vi "GUI_Bella_Control_Center_iP2.vi"() -> ()   [LabVIEW 2020]
uses:
  Shared/GUI_Template/GUI_master/tcp_new_data_event.ctl
  Shared/GUI_Template/GUI_master/tcp new data cluster.ctl
  GUI_TestStand/Fire button.ctl
  Device Drivers/DG645/subVIs/TriggerSource_TypDef.ctl
  <vilib>/Utility/config.llb/Write Key (I32).vi
  <vilib>/Platform/browser.llb/Open URL in Default Browser (string).vi
  <vilib>/Utility/config.llb/NI_LVConfig.lvlib
panel:
  out "got manpar ofi bool data":bool
  out "got manpar ofi data":bool
  out "set expt editor":bool
  in  "Delay.Ch D::10":dbl=-1.631e-06 caption="Delay D" min=-0.1 max=20.0 format="%.4f"
  in  "value6::42":dbl=0.006 caption="PostScanRate" min=0.1 max=1.0 format="%#_3f"
  in  "value5::42":dbl=0.006 caption="1BL-2BL-\nSplitter-Rpcnt" min=-9999999.0 max=9999999.0 format="%#_6p"
  in  "value6::43":bool=TRUE caption="GhostFoil-In"
  in  "value5::43":bool=TRUE caption="1BL-Energy\nMeter-In"
  in  "value4::43":bool=TRUE caption="2BLFoil-In"
  in  "value3::43":bool=TRUE caption="1BLFoil-In"
  in  "value2::43":bool=TRUE caption="ClunkerIn"
  out "CurrentStatus":string
  in  "MoveStage":bool
  in  "Position.Ch1::44":dbl caption="Current Position" min=0.0 max=150.0
  in  "GUIdevice 44":string="STAGE-LT-Megattenuator"
  in  "GUIdevice 43":string="MANPAR-BELLA-OFI-Boolean"
  in  "GUIdevice 42":string="MANPAR-BELLA-OFI"
  out "HPD2 to match HPD":dbl
  in  "Save \ncreenshots":bool
  out "error out":errorcluster
  out "HPD - focus":dbl
  in  "value1::42":dbl=230.0 caption="focus on HPD" min=-9999999.0 max=9999999.0
  in  "value0::43":bool=TRUE caption="SCS"
  in  "Thales.DIAG_CU_Output_Percent_1::37":dbl caption="Amp2 att (%)" min=1.0 max=100.0 step=500.0 format="%.2f"
  in  "GUIdevice 37":string="SVE-LT-Thales"
  in  "Scan":T1(ring)
  in  "LogTable":bool
  in  "New Google\nExpLog for new day?":bool=TRUE
  out "standard output":string
  in  "Create Log":bool caption="LogTable"
  in  "Position.Channel 5::31":T2(ring) caption="FROG foil"
  in  "Position.Channel 2::31":T2(ring) caption="Little Rick"
  in  "Step size 2":dbl=20.0 caption="Step size" min=-22.0 max=22.0
  in  "Position.Axis 4::33":dbl caption="Holy M V F4" min=-100000.0 max=100000.0 step=500.0
  in  "Position.Axis 3::33":dbl caption="Holy M H F3" min=-1000000.0 max=1000000.0 step=500.0
  in  "Position.Axis 2::33":dbl caption="Bessel M3 V F2" min=-100000.0 max=100000.0 step=500.0
  in  "Position.Axis 1::33":dbl caption="Bessel M3 H F1" min=-100000.0 max=100000.0 step=500.0
  in  "GUIdevice 33":string="MCD-PL1-picosOFI1"
  in  "GUIdevice 4":string="STAGE-PL1-Capstage1"
  in  "GUIdevice 31":string="1WIRE-BELLA-Flipper"
  in  "Amplitude.Ch GH::10":dbl=-1.631e-06 caption="Shot Shutter V" min=0.5 max=5.0 format="%.1f"
  in  "Rate (Hz)":dbl=0.3
  in  "Heater Alignment Directions":bool
  in  "Position.Axis 3::15":dbl caption="XY" min=-3.0 max=16.0 format="%.4f"
  in  "Position.Axis 2::15":dbl caption="Y" min=-3.0 max=17.0 format="%.4f"
  in  "Position.Axis 1::15":dbl caption="X" min=-3.0 max=13.0 format="%.4f"
  in  "GUIdevice 24":string="STAGE-HEAT-TL1"
  in  "Encoder position::23":dbl caption="position HPD2" min=0.0 max=600.0 format="%.1f"
  in  "position::3":dbl caption="position HPD" min=0.0 max=600.0 format="%.1f"
  in  "GUIdevice 23":string="STAGE-HPD-Far"
  in  "GUIdevice 22":string="MANPAR-BELLA-FireCont"
  in  "Allow Fire Continues":bool
  out "Fire continues Indicator":bool caption="firing"
  in  "Fire Button":T3=TRUE
  in  "Trigger.Source::10":T4 caption="SRS Trigger Mode"
  out "Absolute discharge timing":dbl caption="delay from pk" format="%#.3p"
  in  "Delay.Ch E::17":dbl caption="Timing box" min=-0.1 max=0.1 format="%.3p"
  in  "value0::22":bool caption="Fire continuosly"
  in  "GUIdevice 15":string="MCD-HEAT-ESP1"
  in  "GUIdevice 17":string="DDG-AA-SRS0"
  out "error IO 2":errorcluster
  out "fire::10":string
  out "tcp data event":T5
  in  "UDP error message":string
  in  "GUIdevice 13":string="DDG-AA-SRS2"
  in  "GUIdevice 2":string="MANPAR-BELLA-General"
  in  "GUIdevice 10":string="DDG-AA-ShotCntrl"
  in  "GUIdevice 1":string="HEX-PL1-1"
  in  "GUIdevice 3":string="STAGE-HPD-Tel"
  in  "Position.Axis 1::9":dbl caption="Comp1 Translation" min=-50.0 max=50.0 format="%.3f"
  in  "GUIdevice 9":string="STAGE-1BL-Compression"
  in  "stop":bool
  # "BELLA ip2 CONTROL CENTER"
  # "Scan"
  # "Safety"
  # "needs manpar-bella-ofi on\nMANPAR-BELLA-OFI-Boolean"
  # "Discharge timing (s)"
  # "1wire"
  # "DG"
  # "PICOS"
  # "Heater timing (s)"
  # "HPD Stage"
  # "Megattenuator Stage"
  # "Attenuate"
  # "OUT"
  # "IN"
  # "Compressor"
  # "Heater Alignment"
  # "Heat ESP0"
  # "Heat ESP1"
  # "Heat Pico"
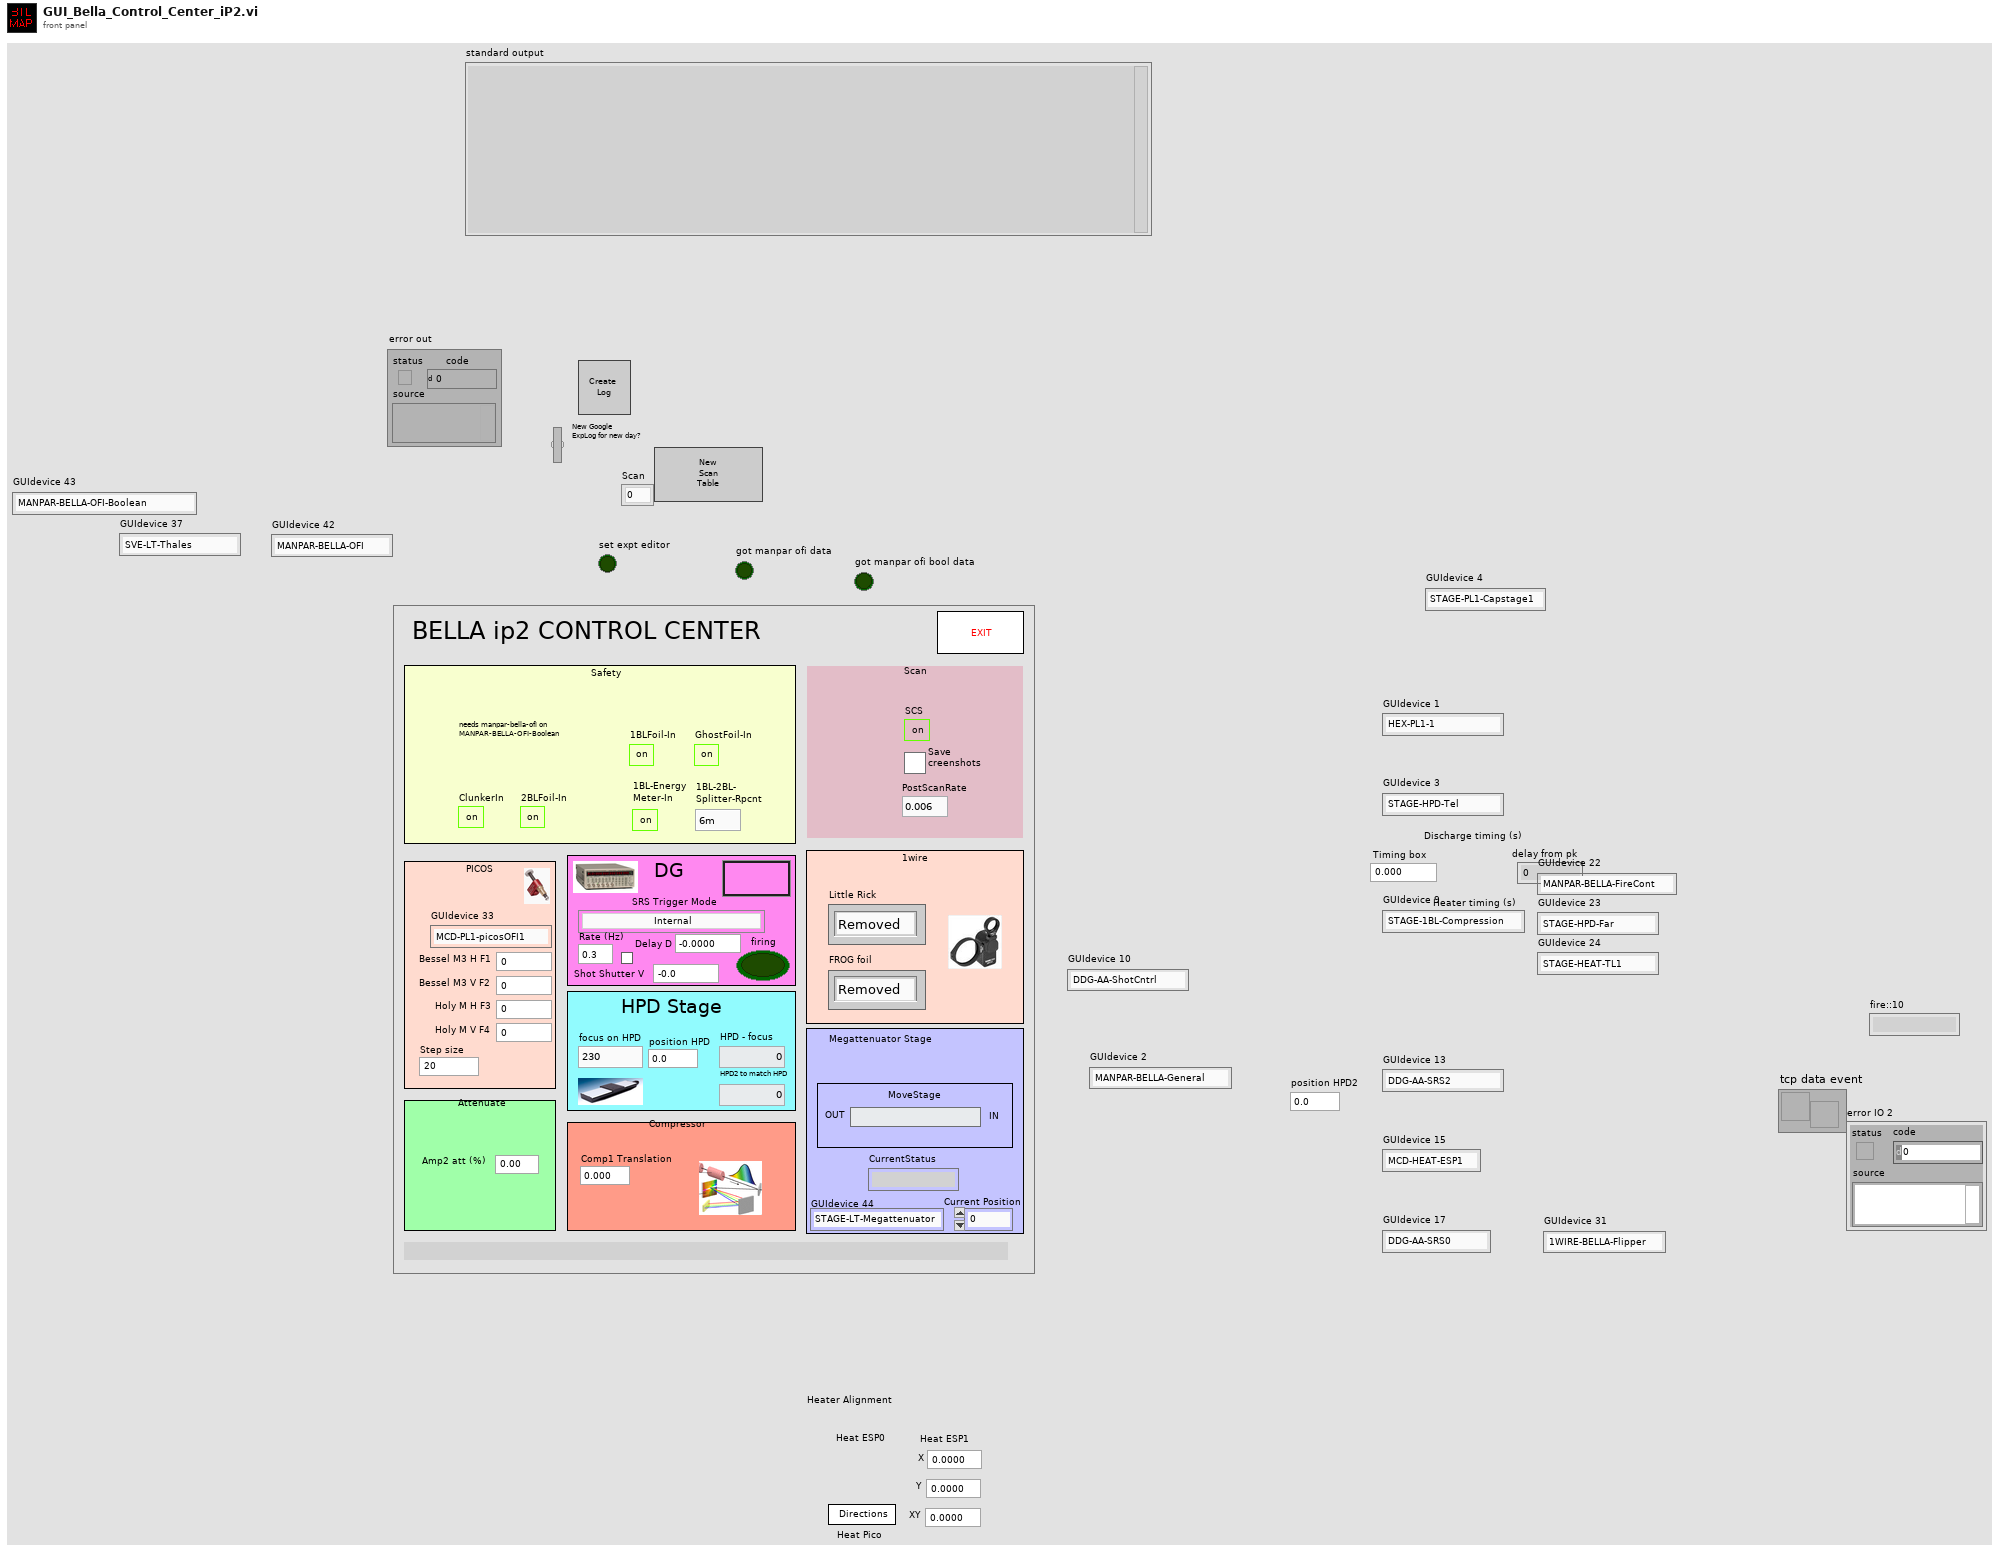
[diagram p1: front panel]
types:
  T1 = enum16{"0", "1", "2", "3", "4", "5", "6", "7", "8", "9", "10", "11", "12", "13", "14", "15", "16", "17", "18", "19", "20", "21", "22", "23", "24", "25", "26", "27", "28", "29", "30", "31", "32", "33", "34", "35", "36", "37", "38", "39", "40", "41", "42", "43", "44", "45", "46", "47", "48", "49", "50", "51", "52", "53", "54", "55", "56", "57", "58", "59", "60", "61", "62", "63", "64", "65", "66", "67", "68", "69", "70", "71", "72", "73", "74", "75", "76", "77", "78", "79", "81", "82", "83", "84", "85", "86", "87", "88", "89", "90", "91", "92", "93", "94", "95", "96", "97", "98", "99", ""}
  T2 = enum16{"Removed", "Inserted", "Unknown", "Moving"}
  T3 = typedef "Fire button.ctl" = bool
  T4 = typedef "TriggerSource_TypDef.ctl" = enum16{"Internal", "External rising edges", "External falling edges", "Single shot external rising edges", "Single shot external falling edges", "Single shot", "Line"}
  T5 = typedef "tcp_new_data_event.ctl" = refnum<user-event>
  T6 = typedef "tcp new data cluster.ctl" = cluster{"EventEnum":enum16{"new data", "connection status update"}, "Device name":string}
  T7 = enum32{"invalid app kind", "Development System", "Run Time System", "Student Edition", "Embedded LabVIEW", "Evaluation", "Custom"}
  T8 = enum32{"Invalid", "Standard", "Closed", "Hidden", "Minimized", "Maximized"}
  T9 = enum8{"Enabled", "Disabled", "Disabled and Grayed Out"}
  T10 = typedef "imagedata.ctl" = cluster{"image type":i32, "image depth":i32, "image":u8[], "mask":u8[], "colors":u32[], "Rectangle":cluster{"left":i16, "top":i16, "right":i16, "bottom":i16}}
  T11 = typedef "NI_LVConfig.lvlib/Config Data RefNum.ctl" = refnum<k1>
  T12 = cluster{"Core":cluster{"Current VI Reference":refnum<vi>, "Close Panel on Exit?":bool}, "Heater timing offset":dbl, "Discharge timing offset":dbl, "Jet trigger":bool, "Tik1":u32, "Tik2":u32, "Fire Continues Allowed":bool}
  T13 = cluster{"Current VI Reference":refnum<vi>, "Close Panel on Exit?":bool}
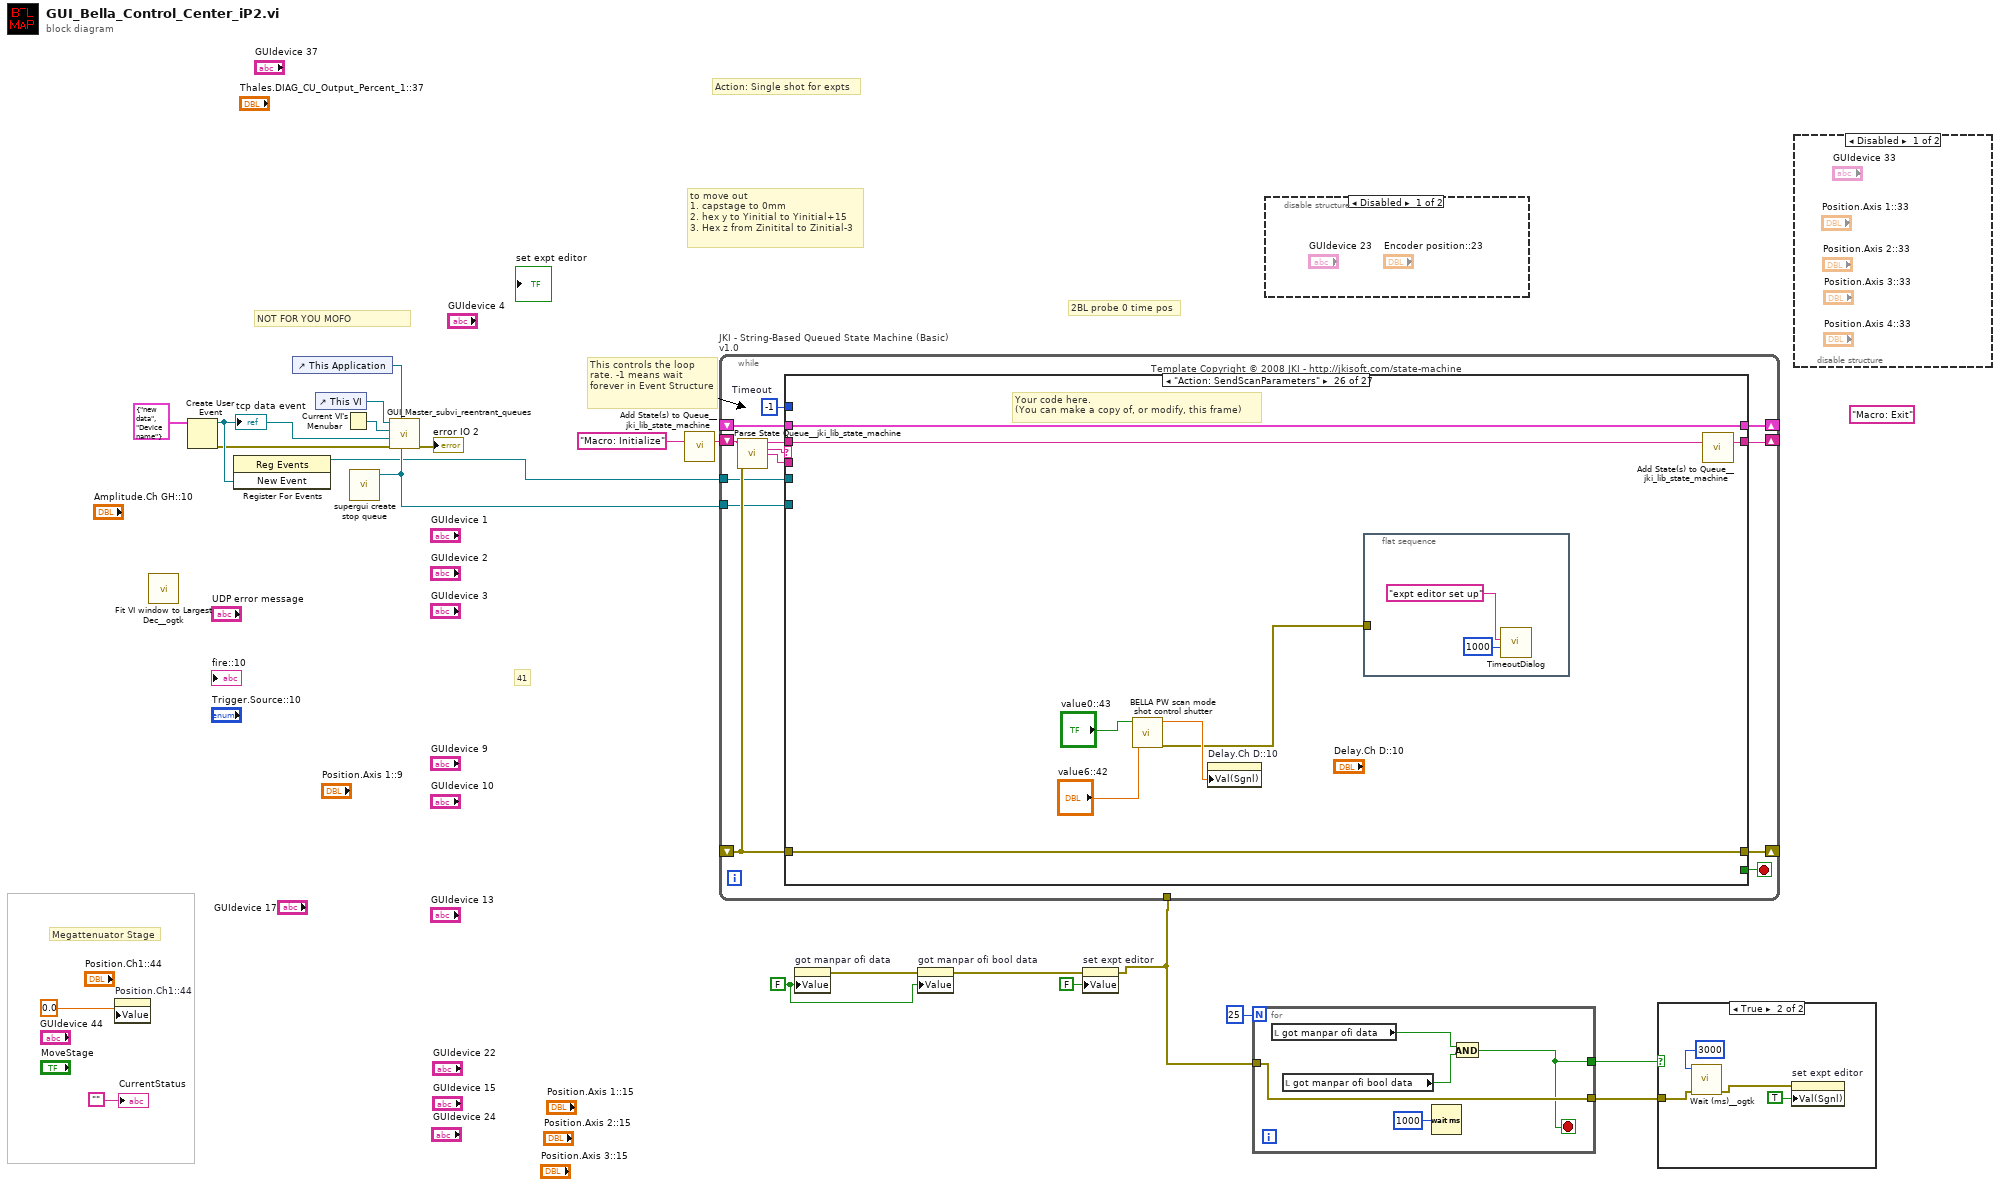
[diagram p0: block diagram]
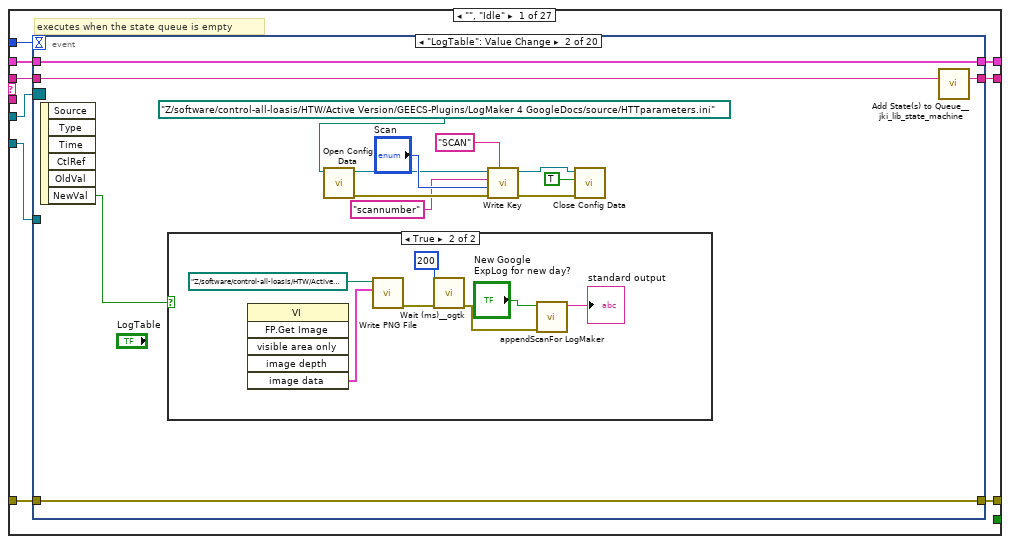
[diagram p5: hidden frame]
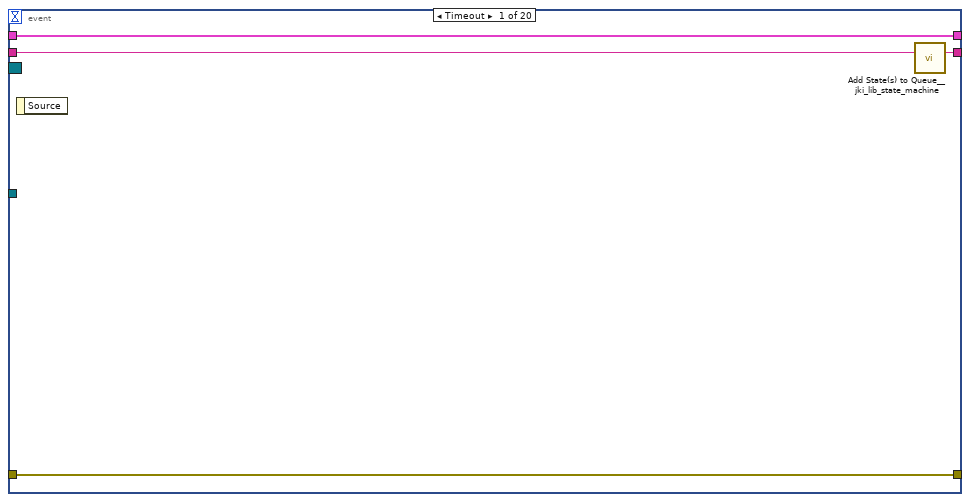
[diagram p6: hidden frame]
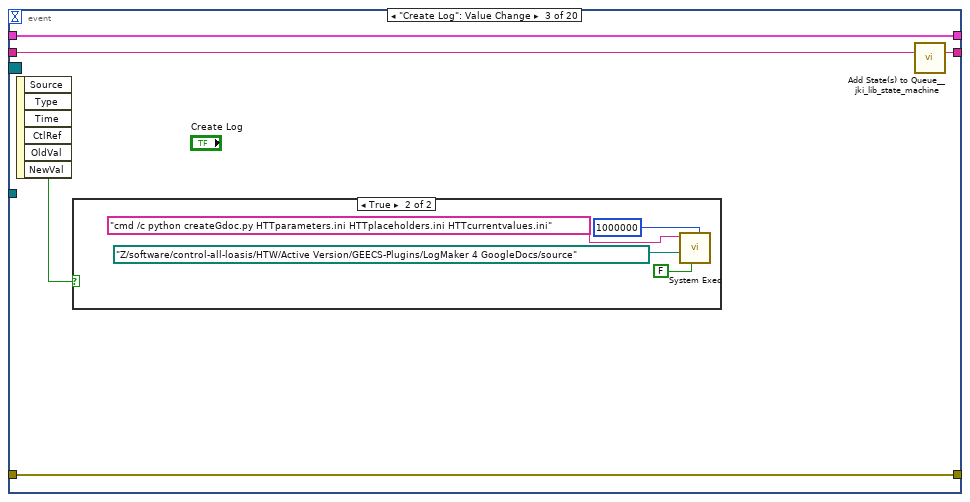
[diagram p8: hidden frame]
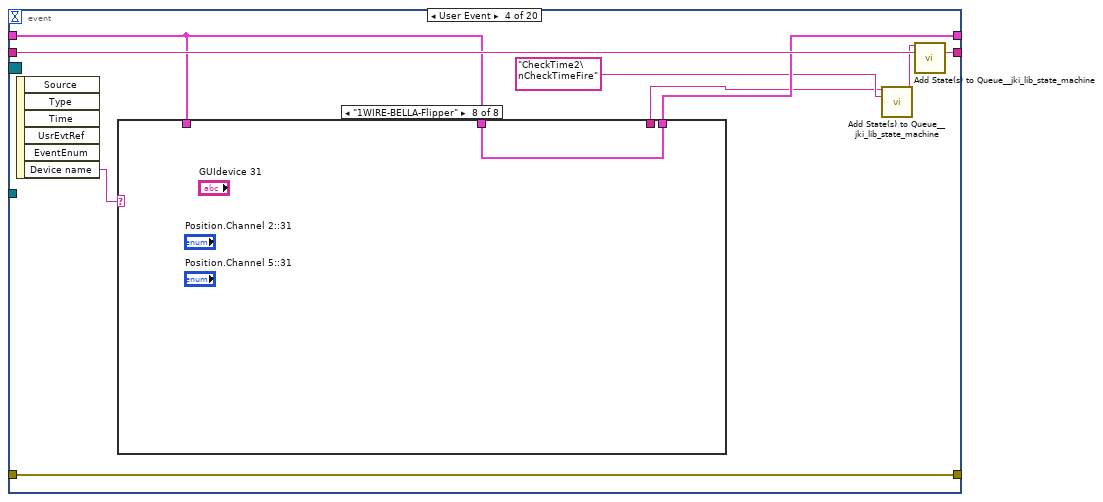
[diagram p10: hidden frame]
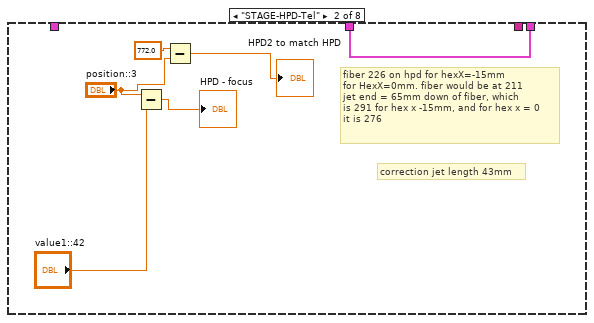
[diagram p12: hidden frame]
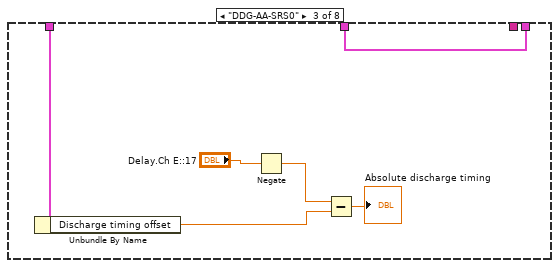
[diagram p13: hidden frame]
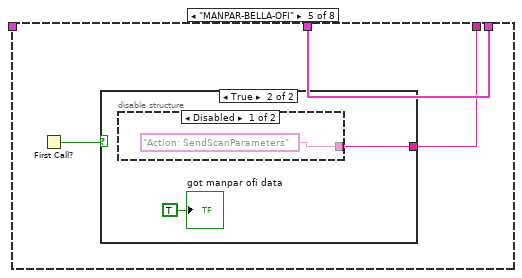
[diagram p15: hidden frame]
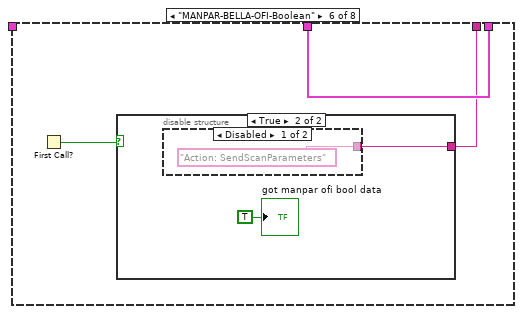
[diagram p18: hidden frame]
diagram:
  w5 = FALSE ("got manpar ofi data")
  (unwired) "Macro: Exit"
  # "41"
  # "Megattenuator Stage"
  # "2BL probe 0 time pos"
  # "Action: Single shot for expts"
  # "to move out\n1. capstage to 0mm\n2. hex y to Yinitial to Yinitial+15\n3. Hex z from Zinitital to Zinitial-3"
  # "This controls the loop rate. -1 means wait forever in Event Structure"
  # "NOT FOR YOU MOFO"
  n1 = property on="Position.Ch1::44" class="DigNum (strict)"("Value"=0.0 ("Position.Ch1::44")) -> ()  [unwired: 2 in, 2 out]
  n2 = call <userlib>:"Fit VI window to Largest Dec__ogtk.vi"() -> ()  [unwired: 6 in, 2 out]
  n3 = Create User Event(user event datatype=T6 {"EventEnum"=enum."new data", "Device name"="Device name"} ("New Event")) -> (user event=w20:refnum<user-event>, error out=w19:errorcluster)  [unwired: 1 in]
  "tcp data event" <- w20
  n4 = register-events(w20) -> (reference out=w11:refnum<event-registration>)  [unwired: 2 in, 1 out]
  n5 = control-ref of="This Application"() -> (w21:refnum<vi>)
  n6 = control-ref of="This VI"() -> (w15:refnum<vi>)
  n7 = Current VI's Menubar() -> (w17:refnum<k9>)
  n8 = call "supergui create stop queue.vi"() -> ("STOP Queue out"=w12:refnum<queue>)  [unwired: 11 in]
  n9 = call "GUI_Master_subvi_reentrant_queues.vi"("STOP Queue in"=w12, "This Application"=w21, "error in (no error)"=w19, "tcp data event"=w20, "Caller menu reference"=w17, "Caller VI ref"=w15) -> ("error out"=→"error IO 2":errorcluster)  [unwired: 5 in]
  n10 = call <vilib>:"Add State(s) to Queue__jki_lib_state_machine.vi"("State(s) in (\"\")"="Macro: Initialize") -> ("States Out"=w13:string)  [unwired: 14 in]
  n11 = property on="got manpar ofi data" class="Bool (strict)"("Value"=w5) -> (error out=w6:errorcluster)  [unwired: 2 in, 1 out]
  n12 = property on="got manpar ofi bool data" class="Bool (strict)"(error in=w6, "Value"=w5) -> (error out=w7:errorcluster)  [unwired: 1 in, 1 out]
  n13 = property on="set expt editor" class="Bool (strict)"(error in=w7, "Value"=FALSE ("set expt editor")) -> (error out=w4:errorcluster)  [unwired: 1 in, 1 out]
  n14 = while "JKI - String-Based Queued State Machine (Basic) v1.0" {
    shift-right: [w27] -> _
    shift-left: _ -> [w26]
    shift-right: [w30] -> _
    shift-left: _ -> [w24]
    shift-right: [w29] -> _
    shift-left: w13 -> [w31]
    tunnel: w11 -> [w23]
    tunnel: w12 -> [w22]
    tunnel: w4 -> [_]
    stop <- w28 stop-if-true
    w25 = -1  # Timeout
    # "Template Copyright © 2008 JKI - http://jkisoft.com/state-machine"
    n15 = call <vilib>:"Parse State Queue__jki_lib_state_machine.vi"("State Queue"=w31, "Error In (no error)"=w24) -> ("Remaining States"=w33:string, "Current State"=w34:string, "Arguments"=w32:string)  [unwired: 11 in]
    n16 = case shown="\"Action: SendScanParameters\"" w34 {
      selector: w34 -> [_ _ w279 _ _ _ _ _ _ _ _ _ _ _ _ _ _ _ _ _ _ _ _ _ _ _ _]
      tunnel: w33 -> [w43 w278 w283 w301 w307 w312 w316 w327 w333 w337 w341 w347 w358 w384 w389 w402 w406 w412 w421 w458 w469 w481 w493 w502 w506 w514 w521]
      tunnel: w32 -> [_ _ _ _ _ _ _ _ _ _ _ w342 w352 _ _ _ _ _ _ _ _ _ _ _ _ _ _]
      tunnel: w26 -> [w41 w275 w281 w292 w304 w310 w313 _ w328 w334 w339 w345 w354 w381 w386 w399 w403 w409 w418 w446 w465 w475 w490 w500 w503 w511 w518]
      tunnel: [w40 w276 w285 w298 errorcluster {"status"=FALSE, "code"=0, "source"=""} ("error out") w309 w314 w324 w329 w335 w338 w343 w355 w382 w387 w400 w404 w410 w419 w456 w463 w470 w491 w497 w504 w512 w519] -> w30
      tunnel: w24 -> [w39 w276 w284 w298 w303 w309 w314 w324 w330 w335 w338 w344 w356 w382 w387 w400 w404 w410 w419 w456 w467 w471 w491 w498 w504 w512 w519]
      tunnel: [w42 w277 w282 w300 w306 w311 w315 w326 w332 w336 w340 w346 w357 w383 w388 w401 w405 w411 w420 w457 w468 w480 w492 w501 w505 w513 w520] -> w29
      tunnel: [_ _ _ _ _ TRUE _ _ _ _ _ _ _ _ _ _ _ _ _ _ _ _ _ _ _ _ _] -> w28
      tunnel: [w35 w275 w281 w299 w304 w310 w313 w325 w328 w334 w339 w345 w354 w381 w386 w399 w403 w409 w418 w455 w465 w474 w489 w500 w503 w511 w518] -> w27
      tunnel: w25 -> [w38 _ _ _ _ _ _ _ _ _ _ _ _ _ _ _ _ _ _ _ _ _ _ _ _ _ _]
      tunnel: w23 -> [w37 _ _ _ _ _ _ _ _ _ _ _ _ _ _ _ _ _ _ _ _ _ _ _ _ _ _]
      tunnel: w22 -> [w36 _ _ _ _ _ _ _ _ _ _ _ _ _ _ w391 _ _ _ _ _ _ _ _ _ _ _]
      frame "", "Idle" {
        # "executes when the state queue is empty"
        n17 = event shown="[1] \"LogTable\": Value Change" {
          selector: w37 -> [_ _ _ _ _ _ _ _ _ _ _ _ _ _ _ _ _ _ _ _]
          dyn-events: _ -> [_ _ _ _ _ _ _ _ _ _ _ _ _ _ _ _ _ _ _ _]
          timeout: w38 -> [_ _ _ _ _ _ _ _ _ _ _ _ _ _ _ _ _ _ _ _]
          tunnel: w43 -> [w47 w61 w73 w86 w122 w124 w129 w139 w149 w159 w169 w179 w188 w196 w205 w229 w239 w246 w248 w274]
          tunnel: [w46 w60 w72 w85 w121 w125 w130 w140 w150 w160 w170 w180 w189 w196 w204 w227 w239 w246 w247 w273] -> w42
          tunnel: w41 -> [w44 w58 w70 w82 w119 w127 w132 w142 w152 w162 w172 w182 w191 w195 w207 w231 w240 w245 w255 w271]
          tunnel: [w45 w59 w71 w84 w120 w126 w131 w141 w151 w161 w171 w181 w190 w193 w210 w230 w238 w244 w254 w272] -> w40
          tunnel: w39 -> [w45 w59 w71 w84 w120 w126 w131 w141 w151 w161 w171 w181 w190 w194 w209 w230 w238 w244 w254 w272]
          tunnel: [w44 w58 w70 w81 w119 w127 w132 w142 w152 w162 w172 w182 w191 w195 w208 w231 w240 w245 w255 w271] -> w35
          tunnel: w36 -> [_ _ _ _ _ _ _ _ _ _ _ _ _ _ _ _ _ _ _ _]
          event Timeout {
            n18 = event-data() -> ()  [unwired: 1 in, 1 out]
            n19 = call <vilib>:"Add State(s) to Queue__jki_lib_state_machine.vi"("State(s) in (\"\")"=w47) -> ("States Out"=w46:string)  [unwired: 14 in]
          }
          event "LogTable": Value Change {
            n20 = event-data() -> ("NewVal"=w48:bool)  [unwired: 1 in, 5 out]
            n21 = case shown="True" w48 {
              frame False {
              }
              frame True {
                n22 = invoke class="VI" method="FP.Get Image"() -> ("image data"=w68:T10)  [unwired: 6 in, 5 out]
                n23 = call <vilib>:"Write PNG File.vi"("image data"=w68, "path to PNG file"=path "Z:/software/control-all-loasis/HTW/Active Version/GEECS-Plugins/LogMaker 4 GoogleDocs/source/frontpanel.png" ("report file path")) -> ("error out"=w63:errorcluster)  [unwired: 8 in, 1 out]
                n24 = call <userlib>:"Wait (ms)__ogtk.vi"("error in (no error)"=w63, "milliseconds to wait"=u32 200 ("millisecond timer value")) -> ("error out"=w62:errorcluster)  [unwired: 8 in, 1 out]
                n25 = call "appendScanFor LogMaker.vi"("error in (no error)"=w62, "New Google\nExpLog for new day?"="New Google\nExpLog for new day?") -> ("standard output"=→"standard output":string)  [unwired: 9 in]
              }
            }
            n26 = call <vilib>:"Open Config Data.vi"("configuration file path"=path "Z:/software/control-all-loasis/HTW/Active Version/GEECS-Plugins/LogMaker 4 GoogleDocs/source/HTTparameters.ini") -> ("error out"=w55:errorcluster, "refnum"=w53:T11)  [unwired: 8 in, 1 out]
            n27 = call-poly <vilib>:"Write Key.vi"("section"="SCAN", "error in (no error)"=w55, "value"="Scan", "key"="scannumber", "refnum"=w53) -> ("error out"=w56:errorcluster, "refnum out"=w54:T11)  [unwired: 4 in, 1 out]
            n28 = call <vilib>:"Close Config Data.vi"("error in (no error)"=w56, "write file if changed (T)"=TRUE, "refnum"=w54) -> ()  [unwired: 7 in, 2 out]
            n29 = call <vilib>:"Add State(s) to Queue__jki_lib_state_machine.vi"("State(s) in (\"\")"=w61) -> ("States Out"=w60:string)  [unwired: 14 in]
          }
          event "Create Log": Value Change {
            n30 = event-data() -> ("NewVal"=w69:bool)  [unwired: 1 in, 5 out]
            n31 = case shown="True" w69 {
              frame False {
              }
              frame True {
                n32 = call <vilib>:"System Exec.vi"("expected output size  (4096)"=u32 1000000, "run minimized? (F)"=FALSE, "working directory"=path "Z:/software/control-all-loasis/HTW/Active Version/GEECS-Plugins/LogMaker 4 GoogleDocs/source", "command line"="cmd /c python createGdoc.py HTTparameters.ini HTTplaceholders.ini HTTcurrentvalues.ini") -> ()  [unwired: 4 in, 4 out]
              }
            }
            n33 = call <vilib>:"Add State(s) to Queue__jki_lib_state_machine.vi"("State(s) in (\"\")"=w73) -> ("States Out"=w72:string)  [unwired: 14 in]
          }
          event User Event {
            n34 = event-data() -> ("Device name"=w83:string)  [unwired: 1 in, 5 out]
            n35 = case shown="\"1WIRE-BELLA-Flipper\"" w83 {
              tunnel: w82 -> [_ _ w96 _ _ _ _ _]
              tunnel: w82 -> [w87 w93 w94 w100 w103 w109 w116 w117]
              tunnel: [w87 w93 w94 w100 w103 w109 w116 w117] -> w81
              tunnel: [_ _ _ _ w102 w108 "Check Megattenuator Stage Status" ("State(s) in Front (\"\")") _] -> w78
              frame "False", Default {
              }
              frame "STAGE-HPD-Tel" {
                # "correction jet length 43mm"
                # "fiber 226 on hpd for hexX=-15mm\nfor HexX=0mm. fiber would be at 211\njet end = 65mm down of fiber, which\nis 291 for hex x -15mm, and for hex x = 0\nit is 276"
                n36 = Subtract(x="position::3", y="value1::42") -> (x-y=→"HPD - focus":dbl)
                n37 = Subtract(x=772.0 ("y"), y="position::3") -> (x-y=→"HPD2 to match HPD":dbl)
              }
              frame "DDG-AA-SRS0" {
                n38 = Unbundle By Name(w96) -> ("Discharge timing offset"=w95:dbl)
                n39 = Negate(x="Delay.Ch E::17") -> (-x=w97:dbl)
                n40 = Subtract(x=w97, y=w95) -> (x-y=→"Absolute discharge timing":dbl)
              }
              frame "STAGE-2BL-ProbeDelay" {
              }
              frame "MANPAR-BELLA-OFI" {
                n41 = First Call?() -> (First Call?: T/F=w101:bool)
                n42 = case shown="True" w101 {
                  tunnel: [_ w105] -> w102
                  frame False {
                  }
                  frame True {
                    n43 = disable-structure shown="Disabled" {
                      disable-tunnel: ["Action: SendScanParameters" ("State(s) in Front (\"\")") _] -> w105
                      frame Disabled {
                      }
                      frame Enabled {
                      }
                    }
                    "got manpar ofi data" <- TRUE ("got manpar ofi data")
                  }
                }
              }
              frame "MANPAR-BELLA-OFI-Boolean" {
                n44 = First Call?() -> (First Call?: T/F=w107:bool)
                n45 = case shown="True" w107 {
                  tunnel: [_ w111] -> w108
                  frame False {
                  }
                  frame True {
                    n46 = disable-structure shown="Disabled" {
                      disable-tunnel: ["Action: SendScanParameters" ("State(s) in Front (\"\")") _] -> w111
                      frame Disabled {
                      }
                      frame Enabled {
                      }
                    }
                    "got manpar ofi bool data" <- TRUE ("got manpar ofi bool data")
                  }
                }
              }
              frame "STAGE-LT-Megattenuator" {
                n47 = property on="Position.Ch1::44" class="DigNum (strict)"() -> ("Caption.FontStrike"=w113:bool)  [unwired: 2 in, 2 out]
                n48 = Not(x=w113) -> (.not. x?=w114:bool)
                n49 = property on="MoveStage" class="Bool (strict)"("Visible"=w114) -> ()  [unwired: 2 in, 2 out]
                n50 = property on="CurrentStatus" class="Str"("Visible"=w114) -> ()  [unwired: 2 in, 2 out]
              }
              frame "1WIRE-BELLA-Flipper" {
              }
            }
            n51 = call <vilib>:"Add State(s) to Queue__jki_lib_state_machine.vi"("State(s) in Front (\"\")"=w78, "State(s) in (\"\")"="CheckTime2\nCheckTimeFire" ("State(s) in Front (\"\")")) -> ("States Out"=w79:string)  [unwired: 13 in]
            n52 = call <vilib>:"Add State(s) to Queue__jki_lib_state_machine.vi"("State(s) in Front (\"\")"=w79, "State(s) in (\"\")"=w86) -> ("States Out"=w85:string)  [unwired: 13 in]
          }
          event "stop": Value Change {
            # "Exit Button Value Change (pressed) Event\n(this executes Macro: Exit to terminate the VI)"
            n53 = event-data() -> ()  [unwired: 1 in, 6 out]
            n54 = call <vilib>:"Add State(s) to Queue__jki_lib_state_machine.vi"("State(s) in Front (\"\")"="Macro: Exit", "State(s) in (\"\")"=w122) -> ("States Out"=w121:string)  [unwired: 13 in]
          }
          event Value Change {
            n55 = event-data() -> ()  [unwired: 1 in, 6 out]
            n56 = call <vilib>:"Add State(s) to Queue__jki_lib_state_machine.vi"("State(s) in Front (\"\")"="Action: Fire" ("State(s) in Front (\"\")"), "State(s) in (\"\")"=w124) -> ("States Out"=w125:string)  [unwired: 13 in]
          }
          event "value0::43", "value6::42": Value Change {
            n57 = event-data() -> ()  [unwired: 1 in, 6 out]
            n58 = call <vilib>:"Add State(s) to Queue__jki_lib_state_machine.vi"("State(s) in Front (\"\")"="Action: SendScanParameters" ("State(s) in Front (\"\")"), "State(s) in (\"\")"=w129) -> ("States Out"=w130:string)  [unwired: 13 in]
          }
          event "value2::43": Value Change {
            n59 = event-data() -> ()  [unwired: 1 in, 6 out]
            n60 = local read "GUIdevice 43"() -> (w133:string)
            n61 = Select(t="on", s="value2::43", f="off") -> (s? t:f=w138:string)
            n62 = call "DefaultValue_Variable_MC.vi"("Variable In"="value2", "Default Value"=w138, "Device In"=w133) -> ()  [unwired: 1 in]
            n63 = call <vilib>:"Add State(s) to Queue__jki_lib_state_machine.vi"("State(s) in (\"\")"=w139) -> ("States Out"=w140:string)  [unwired: 14 in]
          }
          event "value3::43": Value Change {
            n64 = event-data() -> ()  [unwired: 1 in, 6 out]
            n65 = local read "GUIdevice 43"() -> (w144:string)
            n66 = Select(t="on", s="value3::43", f="off") -> (s? t:f=w148:string)
            n67 = call "DefaultValue_Variable_MC.vi"("Variable In"="value3", "Default Value"=w148, "Device In"=w144) -> ()  [unwired: 1 in]
            n68 = call <vilib>:"Add State(s) to Queue__jki_lib_state_machine.vi"("State(s) in (\"\")"=w149) -> ("States Out"=w150:string)  [unwired: 14 in]
          }
          event "value4::43": Value Change {
            n69 = event-data() -> ()  [unwired: 1 in, 6 out]
            n70 = local read "GUIdevice 43"() -> (w154:string)
            n71 = Select(t="on", s="value4::43", f="off") -> (s? t:f=w158:string)
            n72 = call "DefaultValue_Variable_MC.vi"("Variable In"="value4", "Default Value"=w158, "Device In"=w154) -> ()  [unwired: 1 in]
            n73 = call <vilib>:"Add State(s) to Queue__jki_lib_state_machine.vi"("State(s) in (\"\")"=w159) -> ("States Out"=w160:string)  [unwired: 14 in]
          }
          event "value5::43": Value Change {
            n74 = event-data() -> ()  [unwired: 1 in, 6 out]
            n75 = local read "GUIdevice 43"() -> (w164:string)
            n76 = Select(t="on", s="value5::43", f="off") -> (s? t:f=w168:string)
            n77 = call "DefaultValue_Variable_MC.vi"("Variable In"="value5", "Default Value"=w168, "Device In"=w164) -> ()  [unwired: 1 in]
            n78 = call <vilib>:"Add State(s) to Queue__jki_lib_state_machine.vi"("State(s) in (\"\")"=w169) -> ("States Out"=w170:string)  [unwired: 14 in]
          }
          event "value6::43": Value Change {
            n79 = event-data() -> ()  [unwired: 1 in, 6 out]
            n80 = local read "GUIdevice 43"() -> (w174:string)
            n81 = Select(t="on", s="value6::43", f="off") -> (s? t:f=w178:string)
            n82 = call "DefaultValue_Variable_MC.vi"("Variable In"="value6", "Default Value"=w178, "Device In"=w174) -> ()  [unwired: 1 in]
            n83 = call <vilib>:"Add State(s) to Queue__jki_lib_state_machine.vi"("State(s) in (\"\")"=w179) -> ("States Out"=w180:string)  [unwired: 14 in]
          }
          event "value5::42": Value Change {
            n84 = event-data() -> ()  [unwired: 1 in, 6 out]
            n85 = Number To Fractional String(number="value5::42", precision (6)=i16 4) -> (F-format string=w184:string)  [unwired: 2 in]
            n86 = call "DefaultValue_Variable_MC.vi"("Variable In"="value5", "Default Value"=w184, "Device In"="GUIdevice 42") -> ()  [unwired: 1 in]
            n87 = call <vilib>:"Add State(s) to Queue__jki_lib_state_machine.vi"("State(s) in (\"\")"=w188) -> ("States Out"=w189:string)  [unwired: 14 in]
          }
          event "Heater Alignment Directions": Value Change {
            n88 = event-data() -> ()  [unwired: 1 in, 6 out]
            n89 = case shown="True" "Heater Alignment Directions" {
              tunnel: w194 -> [w197 w200]
              tunnel: [w197 w199] -> w193
              frame False {
              }
              frame True {
                n90 = call-poly <vilib>:"Open URL in Default Browser.vi"("error in (no error)"=w200, "URL"="https://docs.google.com/document/d/1RMZp6W8Kkog2nkTymSjyZ2bh9D7Vo4bxhvGgn3Ut4KE/edit") -> ("error out"=w199:errorcluster)  [unwired: 4 in, 1 out]
              }
            }
          }
          event "Allow Fire Continues": Value Change {
            n91 = event-data() -> ()  [unwired: 1 in, 6 out]
            n92 = Unbundle By Name(w207) -> ("Fire Continues Allowed"=w206:bool)
            n93 = case shown="True" "Allow Fire Continues" {
              tunnel: [w211 w218] -> w210
              tunnel: "Allow Fire Continues" -> [_ w217]
              tunnel: w209 -> [w211 w216]
              tunnel: w206 -> [w212 w215]
              tunnel: [w212 w213] -> w202
              tunnel: [_ "Initilize Fire Continues" ("State(s) in Front (\"\")")] -> w201
              frame False {
              }
              frame True {
                n94 = case shown="False" w215 {
                  tunnel: [w224 w225] -> w218
                  tunnel: w217 -> [w223 _]
                  tunnel: w216 -> [w222 w225]
                  tunnel: [w219 FALSE] -> w213
                  frame False {
                    n95 = call "Password"("Enable"=w223, "error in (no error)"=w222) -> ("Password"=w221:string, "error out"=w224:errorcluster)  [unwired: 15 in, 1 out]
                    n96 = Equal?(x=w221, y="fire") -> (x = y?=w219:bool)
                  }
                  frame True {
                  }
                }
              }
            }
            n97 = Bundle By Name(cluster=w207, "Fire Continues Allowed"=w202) -> (w208:T12)
            n98 = call <vilib>:"Add State(s) to Queue__jki_lib_state_machine.vi"("State(s) in Front (\"\")"=w201, "State(s) in (\"\")"=w205) -> ("States Out"=w204:string)  [unwired: 13 in]
          }
          event "set expt editor": Value Change {
            n99 = event-data() -> ()  [unwired: 1 in, 6 out]
            n100 = call <vilib>:"Add State(s) to Queue__jki_lib_state_machine.vi"("State(s) in Front (\"\")"="Action: SendScanParameters" ("State(s) in Front (\"\")"), "State(s) in (\"\")"=w229) -> ("States Out"=w227:string)  [unwired: 13 in]
          }
          event "Step size 2": Value Change {
            n101 = event-data() -> ("NewVal"=w232:dbl)  [unwired: 1 in, 5 out]
            n102 = control-ref of="Position.Axis 1::33"() -> (w237:refnum<vi>)
            n103 = control-ref of="Position.Axis 2::33"() -> (w236:refnum<vi>)
            n104 = control-ref of="Position.Axis 4::33"() -> (w234:refnum<vi>)
            n105 = control-ref of="Position.Axis 3::33"() -> (w235:refnum<vi>)
            n106 = Build Array(w237, w236, w235, w234) -> (w233:refnum<vi>[])
            n107 = for {
              tunnel: w233 -> [w242] mode=indexing
              tunnel: w232 -> [w241]
              n108 = property on="Property Node" class="DigNum (strict)"(reference=w242, "Increment"=w241) -> ()  [unwired: 1 in, 2 out]
            }
          }
          event Value Change {
            n109 = event-data() -> ()  [unwired: 1 in, 6 out]
            n110 = property on="value0::22" class="Bool (strict)"("Val(Sgnl)"=FALSE) -> ()  [unwired: 2 in, 2 out]
          }
          event "MoveStage": Value Change {
            n111 = event-data() -> ("OldVal"=w250:bool, "NewVal"=w253:bool)  [unwired: 1 in, 4 out]
            n112 = flat-sequence {
              tunnel: w253 -> [w260]
              tunnel: [w260] -> w252
              tunnel: [w257] -> w251
              tunnel: w250 -> [w256]
              tunnel: [w256] -> w249
              tunnel: w252 -> [w263]
              tunnel: w251 -> [w262]
              tunnel: w249 -> [w261]
              frame #0 {
                n113 = call "PasswordPrompt.vi"() -> ("Please enter password below 2"=w259:string)  [unwired: 11 in]
                n114 = Equal?(x=w259, y="l0dat&srv!") -> (x = y?=w257:bool)
              }
              frame #1 {
                n115 = case shown="True" w262 {
                  tunnel: w263 -> [_ w266]
                  tunnel: w261 -> [w264 _]
                  frame False {
                    n116 = call "Display Message to User"("Message"="Wrong Password") -> ()  [unwired: 9 in, 2 out]
                    n117 = property on="MoveStage" class="Bool (strict)"("Value"=w264) -> ()  [unwired: 2 in, 2 out]
                  }
                  frame True {
                    n118 = case shown="True" w266 {
                      frame False {
                        n119 = property on="Position.Ch1::44" class="DigNum (strict)"("Val(Sgnl)"=150.0 ("Value (Signaling)")) -> ()  [unwired: 2 in, 2 out]
                      }
                      frame True {
                        n120 = property on="Position.Ch1::44" class="DigNum (strict)"("Val(Sgnl)"=0.5 ("Value (Signaling)")) -> ()  [unwired: 2 in, 2 out]
                      }
                    }
                    n121 = property on="MoveStage" class="Bool (strict)"("Value"=w266) -> ()  [unwired: 2 in, 2 out]
                  }
                }
              }
            }
            n122 = call <vilib>:"Add State(s) to Queue__jki_lib_state_machine.vi"("State(s) in (\"\")"=w248) -> ("States Out"=w247:string)  [unwired: 14 in]
          }
          event Panel Close? {
            # "Discard the event because we'll close the front panel ourselves in Macro: Exit"
            # "Close Panel button (pressed) Event\n(this executes Macro: Exit to terminate the VI)"
            n123 = event-data() -> ()  [unwired: 1 in, 1 out]
            n124 = event-data("Discard?"=TRUE) -> ()  [unwired: 1 in, 1 out]
            n125 = call <vilib>:"Add State(s) to Queue__jki_lib_state_machine.vi"("State(s) in Front (\"\")"="Macro: Exit", "State(s) in (\"\")"=w274) -> ("States Out"=w273:string)  [unwired: 13 in]
          }
        }
      }
      frame "---------- Core ----------" {
        # "Do not put any code in this frame.\n(it is a separator no-op)"
        n126 = call <vilib>:"Add State(s) to Queue__jki_lib_state_machine.vi"("State(s) in (\"\")"=w278) -> ("States Out"=w277:string)  [unwired: 14 in]
      }
      frame Default {
        w288 = 42 items=["No error", "Argument error", "Memory is full", "Out of zone", "End of file", "File already open", "Generic file I/O error", "File not found", "File permission error", "Disk is full", "Duplicate path", "Too many files open", "System feature not enabled", "Resource file not found", "Cannot add resource", "Resource not found", "Image not found", "Image memory error", "Pen does not exist", "Config type invalid", "Config token not found", "Config parse error", "Config memory error", "Bad external code format", "Bad external code offset", "External code not present", "Null window", "Destroy window error", "Null menu", "Print aborted", "Bad print record", "Print driver error", "Windows error during printing", "Memory error during printing", "Print dialog error", "Generic print error", "Invalid device refnum", "Device not found", "Device parameter error", "Device unit error", "Cannot open device", "Device call aborted", "Generic error", "Cancelled by user", "Object ID too low", "Object ID too high", "Object not in heap", "Unknown heap", "Unknown object (invalid DefProc)", "Unknown object (DefProc not in table)", "Message out of range", "Invalid (null) method", "Unknown message", "Manager call not supported", "Bad address", "Network operation in progress", "Network operation timed out", "Connection is busy", "Network attribute not supported", "Network error", "Address in use", "System out of memory", "Connection aborted", "Connection refused", "Not connected", "Already connected", "Connection closed", "Initialization error (interapplication manager)", "Bad occurrence", "Wait on unbound occurrence handler", "Occurrence queue overflow", "Datalog type conflict", "Unused", "Unrecognized type (interapplication manager)", "Memory corrupt", "Failed to make temporary DLL", "Old CIN version", "Drag socket not found", "Failed to load drop-object", "Failed to register OLE object", "Failed to release OLE object", "Format specifier type mismatch", "Unknown format specifier", "Too few format specifiers", "Too many format specifiers", "Scan failed", "Newer CIN version", "Error converting to variant", "Runtime menu error", "Password tampered", "Variant attribute not found", "Incompatible variant data type", "Event data is not available", "Event Store is not present", "Occurrence is not found", "Event Queue is not created", "Event info is not available", "Refnum passed is NULL", "Error retrieving Class GUID", "Error retrieving CoClass GUID", "Error retrieving TypeLib GUID.", "Bad built application magic bytes.", "Specific driver is different from the specific driver associated with the Logical Name.", "There is no session opened to the class driver.", "Max Error", "MAX - Error with config objects", "MAX - Error loading configuration", "MAX - Group not supported"]
        # "Current State"
        # "Do not delete, rename, or modify this frame.\n(this is used to capture unhandled states and typos)"
        # "Handle mistyped state name (developer tool)"
        n127 = Format Into String(format string="Software Exception: Unhandled State \"%s\"." ("message"), error in=w284, w279) -> (resulting string=w287:string, error out=w286:errorcluster)  [unwired: 1 in]
        n128 = call <vilib>:"Error Cluster From Error Code.vi"("show call chain? (False)"=TRUE, "error in (no error)"=w286, "error message (\"\")"=w287, "error code (0)"=w288) -> ("error out"=w285:errorcluster)  [unwired: 5 in]
        n129 = call <vilib>:"Add State(s) to Queue__jki_lib_state_machine.vi"("State(s) in (\"\")"=w283) -> ("States Out"=w282:string)  [unwired: 14 in]
      }
      frame "Initialize Core Data" {
        # "Do not delete, rename, or modify this frame.\n(this is used to determine panel behavior on exit)"
        # "originally closed?"
        # "exe?"
        # "If panel starts closed or is an EXE, then close it when we exit"
        n130 = property class="VI"() -> ("Front Panel.Open"=w297:bool)  [unwired: 2 in, 2 out]
        n131 = property class="App"() -> ("App.Kind"=w296:T7)  [unwired: 2 in, 2 out]
        n132 = control-ref of="Current VI Reference"() -> (w290:refnum<vi>)
        n133 = Not(x=w297) -> (.not. x?=w294:bool)
        n134 = Equal?(x=w296, y=T7."Run Time System" ("Application:Kind")) -> (x = y?=w293:bool)
        n135 = Or(x=w294, y=w293) -> (x .or. y?=w291:bool)
        n136 = Bundle By Name(cluster=w292, "Core.Current VI Reference"=w290, "Core.Close Panel on Exit?"=w291) -> (w299:T12)
        n137 = call <vilib>:"Add State(s) to Queue__jki_lib_state_machine.vi"("State(s) in (\"\")"=w301) -> ("States Out"=w300:string)  [unwired: 14 in]
      }
      frame "Error Handler" {
        # "Unhandled Error -- Display it"
        # "Handle any errors here.\nYou can also output any states to clean-up after errors occur"
        # "Clear error"
        n138 = call <vilib>:"General Error Handler.vi"("error in (no error)"=w303) -> ()  [unwired: 10 in, 5 out]
        n139 = call <vilib>:"Add State(s) to Queue__jki_lib_state_machine.vi"("State(s) in Front (\"\")"="/* Post Error States", "State(s) in (\"\")"=w307) -> ("States Out"=w306:string)  [unwired: 13 in]
      }
      frame "Exit" {
        # "Do not put any code in this frame.\n(No errors that occur here will be handled.)"
        n140 = call <vilib>:"Add State(s) to Queue__jki_lib_state_machine.vi"("State(s) in (\"\")"=w312) -> ("States Out"=w311:string)  [unwired: 14 in]
      }
      frame "---------- Data ----------" {
        # "Do not put any code in this frame.\n(It is a separator no-op. You can make a copy of this frame to create a new Data frame)"
        n141 = call <vilib>:"Add State(s) to Queue__jki_lib_state_machine.vi"("State(s) in (\"\")"=w316) -> ("States Out"=w315:string)  [unwired: 14 in]
      }
      frame "Data: Initialize" {
        w317 = FALSE  # Fire Continues Allowed
        w319 = u32 0  # Tik1
        w318 = u32 0  # Tik2
        w320 = FALSE  # Jet trigger
        w321 = 0.0  # Discharge timing offset
        w322 = 0.0  # Heater timing offset
        w323 = T13 {"Current VI Reference"=refnum, "Close Panel on Exit?"=FALSE}  # Core
        # "Data names and types of shift register data are defined by this bundle."
        # "Initialize the shift-register data, here.\n(data names are defined by what you wire into the bundle function)"
        n142 = Bundle("Core"=w323, "Heater timing offset"=w322, "Discharge timing offset"=w321, "Jet trigger"=w320, "Tik1"=w319, "Tik2"=w318, "Fire Continues Allowed"=w317) -> (w325:T12)  [unwired: 1 in]
        n143 = call <vilib>:"Add State(s) to Queue__jki_lib_state_machine.vi"("State(s) in (\"\")"=w327) -> ("States Out"=w326:string)  [unwired: 14 in]
      }
      frame "Data: Cleanup" {
        # "Cleanup any data and references, here.\n(this is called automatically, by the Macro: Exit)"
        n144 = Unbundle By Name(w328) -> ("Core.Current VI Reference"=w331:refnum<vi>)
        n145 = Close Reference(reference=w331, error in (no error)=w330) -> (error out=w329:errorcluster)
        n146 = call <vilib>:"Add State(s) to Queue__jki_lib_state_machine.vi"("State(s) in (\"\")"=w333) -> ("States Out"=w332:string)  [unwired: 14 in]
      }
      frame "---------- UI ----------" {
        # "Do not put any code in this frame.\n(It is a separator no-op. You can make a copy of this frame to create a new UI frame)"
        n147 = call <vilib>:"Add State(s) to Queue__jki_lib_state_machine.vi"("State(s) in (\"\")"=w337) -> ("States Out"=w336:string)  [unwired: 14 in]
      }
      frame "UI: Initialize" {
        # "Initialize the User Interface, here.\n(this is called automatically, by the Macro: Init)"
        n148 = call <userlib>:"Fit VI window to Largest Dec__ogtk.vi"() -> ()  [unwired: 6 in, 2 out]
        n149 = call <vilib>:"Add State(s) to Queue__jki_lib_state_machine.vi"("State(s) in (\"\")"=w341) -> ("States Out"=w340:string)  [unwired: 14 in]
      }
      frame "UI: Cursor Set" {
        # "Argument"
        # "Set and Unset Cursor Busy.\n(Usage: \"UI: Cursor Set >> Busy|Idle\")"
        n150 = case shown="\"Idle\", Default" w342 {
          tunnel: w344 -> [w349 w351]
          tunnel: [w348 w350] -> w343
          frame "Idle", Default {
            n151 = call <vilib>:"Unset Busy.vi"("error in (no error)"=w349) -> ("error out"=w348:errorcluster)  [unwired: 10 in]
          }
          frame "Busy" {
            n152 = call <vilib>:"Set Busy.vi"("error in (no error)"=w351) -> ("error out"=w350:errorcluster)  [unwired: 9 in, 1 out]
          }
        }
        n153 = call <vilib>:"Add State(s) to Queue__jki_lib_state_machine.vi"("State(s) in (\"\")"=w347) -> ("States Out"=w346:string)  [unwired: 14 in]
      }
      frame "UI: Front Panel State" {
        # "Argument"
        # "Set Front Panel Open or Closed\n(Usage: \"UI: Front Panel State >> Open|Close\")"
        n154 = Unbundle By Name(w354) -> ("Core.Current VI Reference"=w353:refnum<vi>)
        n155 = case shown="\"Close\"" w352 {
          tunnel: w356 -> [w362 w375]
          tunnel: [w364 w376] -> w355
          tunnel: w353 -> [w363 w373]
          frame "Open", Default {
            n156 = property class="VI"(reference=w363, error in=w362) -> (reference out=w360:refnum<vi>, error out=w361:errorcluster, "Front Panel.Open"=w359:bool)
            n157 = case shown="False" w359 {
              tunnel: [w367 w370] -> w364
              tunnel: w361 -> [w366 w370]
              tunnel: w360 -> [w365 _]
              frame False {
                n158 = invoke class="VI" method="FP.Open"(reference=w365, error in=w366, "Activate"=TRUE, "State"=T8."Standard") -> (error out=w367:errorcluster)  [unwired: 1 in, 4 out]
              }
              frame True {
              }
            }
          }
          frame "Close" {
            n159 = property class="VI"(reference=w373, error in=w375) -> (reference out=w372:refnum<vi>, error out=w374:errorcluster, "Front Panel.Open"=w371:bool)
            n160 = case shown="True" w371 {
              tunnel: [w377 w380] -> w376
              tunnel: w374 -> [w377 w379]
              tunnel: w372 -> [_ w378]
              frame False {
              }
              frame True {
                n161 = invoke class="VI" method="FP.Close"(reference=w378, error in=w379) -> (error out=w380:errorcluster)  [unwired: 1 in, 2 out]
              }
            }
          }
        }
        n162 = call <vilib>:"Add State(s) to Queue__jki_lib_state_machine.vi"("State(s) in (\"\")"=w358) -> ("States Out"=w357:string)  [unwired: 14 in]
      }
      frame "---------- Macro ----------" {
        # "Do not put any code in this frame.\n(It is a separator no-op. You can make a copy of this frame to create a new Macro frame)"
        n163 = call <vilib>:"Add State(s) to Queue__jki_lib_state_machine.vi"("State(s) in (\"\")"=w384) -> ("States Out"=w383:string)  [unwired: 14 in]
      }
      frame "Macro: Initialize" {
        w385 = "Data: Initialize\nInitialize Core Data\nUI: Initialize\nUI: Front Panel State >> Open\nCheck if Fire continues allowed\nInitilize Fire Continues\nInit:MegattenuatorStage"  # Data: Initialize Initialize Core Data UI: Initialize UI: Front Panel State >> Open Check if Fire continues allowed Initilize Fire Continues Init:MegattenuatorStage
        # "Initialization Macro\n(This is called once, when the VI starts)"
        n164 = call <vilib>:"Add State(s) to Queue__jki_lib_state_machine.vi"("State(s) in Front (\"\")"=w385, "State(s) in (\"\")"=w389) -> ("States Out"=w388:string)  [unwired: 13 in]
      }
      frame "Macro: Exit" {
        # "Exit Macro\n(This is called once, when the VI exits)"
        n165 = Unbundle By Name(w399) -> ("Core.Close Panel on Exit?"=w398:bool)
        n166 = Release Queue(queue=w391, force destroy? (F)=TRUE) -> (error out=w390:errorcluster)  [unwired: 1 in, 2 out]
        n167 = call <vilib>:"Clear Errors.vi"("error in (no error)"=w390) -> ()  [unwired: 5 in, 2 out]
        n168 = Select(t="UI: Front Panel State >> Close", s=w398, f="") -> (s? t:f=w395:string)
        n169 = call <vilib>:"Add State(s) to Queue__jki_lib_state_machine.vi"("State(s) in (\"\")"=w395, "State(s) at Back (\"\")"="Data: Cleanup\nExit") -> ("States Out"=w393:string)  [unwired: 13 in]
        n170 = call <vilib>:"Add State(s) to Queue__jki_lib_state_machine.vi"("State(s) in Front (\"\")"=w393, "State(s) in (\"\")"=w402) -> ("States Out"=w401:string)  [unwired: 13 in]
      }
      frame "---------- New Category ----------" {
        # "Template Separator\n(You can make a copy of, or modify, this frame)"
        n171 = call <vilib>:"Add State(s) to Queue__jki_lib_state_machine.vi"("State(s) in (\"\")"=w406) -> ("States Out"=w405:string)  [unwired: 14 in]
      }
      frame "Check Megattenuator Stage Status" {
        n172 = property on="Position.Ch1::44" class="DigNum (strict)"() -> ("Value"=w407:dbl)  [unwired: 2 in, 2 out]
        n173 = case shown="0, 1" w407 {
          tunnel: ["IN" "Unknown/Moving" "OUT"] -> w408
          frame 0, 1 {
            n174 = property on="MoveStage" class="Bool (strict)"("Value"=TRUE) -> ()  [unwired: 2 in, 2 out]
          }
          frame 2, Default {
          }
          frame 149..151 {
            n175 = property on="MoveStage" class="Bool (strict)"("Value"=FALSE) -> ()  [unwired: 2 in, 2 out]
          }
        }
        n176 = property on="CurrentStatus" class="Str"("Value"=w408) -> ()  [unwired: 2 in, 2 out]
        n177 = call <vilib>:"Add State(s) to Queue__jki_lib_state_machine.vi"("State(s) in (\"\")"=w412) -> ("States Out"=w411:string)  [unwired: 14 in]
      }
      frame "Init:MegattenuatorStage" {
        # "Template Separator\n(You can make a copy of, or modify, this frame)"
        n178 = disable-structure shown="Disabled" {
          frame Disabled {
            n179 = flat-sequence {
              frame #0 {
                n180 = call <vilib>:"Set Busy.vi"("disable click? (T)"=TRUE, "cursor ID"=refnum<k1> refnum) -> ()  [unwired: 8 in, 2 out]
              }
              frame #1 {
                n181 = while {
                  tunnel: [w433] -> w425
                  i -> [w428]
                  stop <- w429 stop-if-true
                  n182 = property on="Position.Ch1::44" class="DigNum (strict)"() -> ("Value"=w433:dbl)  [unwired: 2 in, 2 out]
                  n183 = Equal?(x=50, y=w428) -> (x = y?=w426:bool)
                  n184 = Not Equal?(x=w433, y=0.0) -> (x != y?=w430:bool)
                  n185 = Wait (ms)(milliseconds to wait=u32 100) -> ()  [unwired: 1 out]
                  n186 = Or(x=w430, y=w426) -> (x .or. y?=w429:bool)
                }
                n187 = case shown="0, 1" w425 {
                  tunnel: ["IN" "Unknown" "OUT"] -> w424
                  frame 0, 1 {
                    n188 = property on="MoveStage" class="Bool (strict)"("Value"=TRUE) -> ()  [unwired: 2 in, 2 out]
                  }
                  frame 2, Default {
                    n189 = property on="MoveStage" class="Bool (strict)"("DisabledEnum"=T9."Disabled" ("Disabled")) -> ()  [unwired: 2 in, 2 out]
                  }
                  frame 149..151 {
                    n190 = property on="MoveStage" class="Bool (strict)"("Value"=FALSE) -> ()  [unwired: 2 in, 2 out]
                  }
                }
                n191 = property on="CurrentStatus" class="Str"("Value"=w424) -> ()  [unwired: 2 in, 2 out]
              }
              frame #2 {
                n192 = call <vilib>:"Unset Busy.vi"() -> ()  [unwired: 11 in, 1 out]
              }
            }
          }
          frame Enabled {
          }
        }
        n193 = call <vilib>:"Add State(s) to Queue__jki_lib_state_machine.vi"("State(s) in (\"\")"=w421) -> ("States Out"=w420:string)  [unwired: 14 in]
      }
      frame "CheckTimeFire" {
        # "Your code here.\n(You can make a copy of, or modify, this frame)"
        n194 = Unbundle By Name(w446) -> ("Tik1"=w451:u32)
        n195 = Tick Count (ms)() -> (millisecond timer value=w453:u32)
        n196 = Unbundle By Name(w446) -> ("Fire Continues Allowed"=w443:bool)
        n197 = Reciprocal(x="Rate (Hz)") -> (1/x=w442:dbl)
        n198 = Subtract(x=w453, y=w451) -> (x-y=w454:u32)
        n199 = Multiply(x=1000.0, y=w442) -> (x*y=w441:dbl)
        n200 = Greater?(x=w454, y=w441) -> (0:w449:bool)
        n201 = And(x=w449, y="value0::22") -> (x .and. y?=w445:bool)
        n202 = And(x=w443, y=w445) -> (x .and. y?=w444:bool)
        n203 = case shown="True" w444 {
          tunnel: w453 -> [_ w461]
          tunnel: [w459 w461] -> w452
          tunnel: w451 -> [w459 _]
          tunnel: [_ "Action: Fire" ("State(s) in Front (\"\")")] -> w448
          frame False {
          }
          frame True {
          }
        }
        n204 = Bundle By Name(cluster=w446, "Tik1"=w452) -> (w455:T12)
        n205 = call <vilib>:"Add State(s) to Queue__jki_lib_state_machine.vi"("State(s) in Front (\"\")"=w448, "State(s) in (\"\")"=w458) -> ("States Out"=w457:string)  [unwired: 13 in]
        "Fire continues Indicator" <- "value0::22"
      }
      frame "Initilize Fire Continues" {
        # "Your code here.\n(You can make a copy of, or modify, this frame)"
        n206 = Unbundle By Name(w465) -> ("Fire Continues Allowed"=w464:bool)
        n207 = property on="value0::22" class="Bool (strict)"(error in=w467, "Visible"=w464) -> (error out=w466:errorcluster)  [unwired: 1 in, 1 out]
        n208 = Not(x=w464) -> (.not. x?=w462:bool)
        n209 = property on="Fire continues Indicator" class="Bool (strict)"(error in=w466, "Visible"=w462) -> (error out=w463:errorcluster)  [unwired: 1 in, 1 out]
        n210 = call <vilib>:"Add State(s) to Queue__jki_lib_state_machine.vi"("State(s) in (\"\")"=w469) -> ("States Out"=w468:string)  [unwired: 14 in]
      }
      frame "Check if Fire continues allowed" {
        # "Check if it is allowed computer"
        # "Your code here.\n(You can make a copy of, or modify, this frame)"
        n211 = String To IP() -> (0:w477:u32)  [unwired: 1 in]
        n212 = IP To String(1:TRUE ("dot notation? (F)"), 2:w477) -> (0:w478:string)
        n213 = Equal?(x=w478, y="192.168.14.2") -> (x = y?=w472:bool)
        n214 = Not(x=w472) -> (.not. x?=w473:bool)
        n215 = Bundle By Name(cluster=w475, "Fire Continues Allowed"=w472) -> (w474:T12)
        n216 = property on="Allow Fire Continues" class="Bool (strict)"(error in=w471, "Visible"=w473) -> (error out=w470:errorcluster)  [unwired: 1 in, 1 out]
        n217 = call <vilib>:"Add State(s) to Queue__jki_lib_state_machine.vi"("State(s) in (\"\")"=w481) -> ("States Out"=w480:string)  [unwired: 14 in]
      }
      frame "CheckTime2" {
        # "Your code here.\n(You can make a copy of, or modify, this frame)"
        n218 = Unbundle By Name(w490) -> ("Tik2"=w483:u32)
        n219 = Tick Count (ms)() -> (millisecond timer value=w485:u32)
        n220 = Subtract(x=w485, y=w483) -> (x-y=w488:u32)
        n221 = Greater?(x=w488, y=5000) -> (0:w486:bool)
        n222 = case shown="True" w486 {
          tunnel: w485 -> [_ w496]
          tunnel: [w494 w496] -> w484
          tunnel: w483 -> [w494 _]
          tunnel: [_ "Action: update expt vars\nAction: save screenshot"] -> w482
          frame False {
          }
          frame True {
          }
        }
        n223 = Bundle By Name(cluster=w490, "Tik2"=w484) -> (w489:T12)
        n224 = call <vilib>:"Add State(s) to Queue__jki_lib_state_machine.vi"("State(s) in Front (\"\")"=w482, "State(s) in (\"\")"=w493) -> ("States Out"=w492:string)  [unwired: 13 in]
      }
      frame "Action: Fire" {
        n225 = property on="fire::10" class="Str"(error in=w498, "Val(Sgnl)"="fire>>force" ("Value (Signaling)")) -> (error out=w497:errorcluster)  [unwired: 1 in, 1 out]
        n226 = call <vilib>:"Add State(s) to Queue__jki_lib_state_machine.vi"("State(s) in (\"\")"=w502) -> ("States Out"=w501:string)  [unwired: 14 in]
      }
      frame "Action: update expt vars" {
        # "Your code here.\n(You can make a copy of, or modify, this frame)"
        n227 = call <vilib>:"Add State(s) to Queue__jki_lib_state_machine.vi"("State(s) in (\"\")"=w506) -> ("States Out"=w505:string)  [unwired: 14 in]
      }
      frame "Action: SendScanParameters" {
        # "Your code here.\n(You can make a copy of, or modify, this frame)"
        n228 = call "BELLA PW scan mode shot control shutter.vi"("PostScanRate"="value6::42", "ScanShotControl"="value0::43") -> ("error out"=w507:errorcluster, "delay D to set"=w508:dbl)  [unwired: 8 in]
        n229 = property on="Delay.Ch D::10" class="DigNum (strict)"("Val(Sgnl)"=w508) -> ()  [unwired: 2 in, 2 out]
        n230 = flat-sequence {
          tunnel: w507 -> [_]
          frame #0 {
            n231 = call "TimeoutDialog.vi"("message 2"="expt editor set up" ("message"), "Timeout(ms)"=u32 1000) -> ()  [unwired: 9 in]
          }
        }
        n232 = call <vilib>:"Add State(s) to Queue__jki_lib_state_machine.vi"("State(s) in (\"\")"=w514) -> ("States Out"=w513:string)  [unwired: 14 in]
      }
      frame "Action: save screenshot" {
        # "Your code here.\n(You can make a copy of, or modify, this frame)"
        n233 = case shown="True" "Save \ncreenshots" {
          frame False {
          }
          frame True {
            n234 = invoke class="VI" method="FP.Get Image"() -> ("image data"=w524:T10)  [unwired: 6 in, 5 out]
            n235 = call <vilib>:"Write PNG File.vi"("image data"=w524, "path to PNG file"=path "N:/data/ECS dumps/Logmaker Screenshot/frontpanel.png" ("report file path")) -> ("error out"=→"error out":errorcluster)  [unwired: 8 in, 1 out]
          }
        }
        n236 = call <vilib>:"Add State(s) to Queue__jki_lib_state_machine.vi"("State(s) in (\"\")"=w521) -> ("States Out"=w520:string)  [unwired: 14 in]
      }
    }
  }
  n237 = for {
    N: 25 -> [_]
    tunnel: w4 -> [w527]
    tunnel: [w527] -> w3
    tunnel: [w525] -> w1
    stop <- w525 stop-if-true
    n238 = local read "got manpar ofi data"() -> (w529:bool)
    n239 = local read "got manpar ofi bool data"() -> (w528:bool)
    n240 = Wait (ms)(milliseconds to wait=u32 1000) -> ()  [unwired: 1 out]
    n241 = And(x=w529, y=w528) -> (x .and. y?=w525:bool)
  }
  n242 = disable-structure shown="Disabled" {
    frame Disabled {
    }
    frame Enabled {
    }
  }
  n243 = case shown="True" w1 {
    tunnel: w3 -> [_ w530]
    frame False {
    }
    frame True {
      n244 = call <userlib>:"Wait (ms)__ogtk.vi"("error in (no error)"=w530, "milliseconds to wait"=u32 3000) -> ("error out"=w532:errorcluster)  [unwired: 8 in, 1 out]
      n245 = property on="set expt editor" class="Bool (strict)"(error in=w532, "Val(Sgnl)"=TRUE ("Value (Signaling)")) -> ()  [unwired: 1 in, 2 out]
    }
  }
  n246 = disable-structure shown="Disabled" {
    frame Disabled {
    }
    frame Enabled {
    }
  }
  "CurrentStatus" <- ""
